vi "Disable Radio Buttons.vi"(10 "Array in":variant[](array[variant]), 11 "Controls[]":refnum<vi>[](array[refnum])) -> (3 "Array out":i32[](array[numeric]))   [LabVIEW 2020]
panel:
  out "error out":errorcluster
  in  "error in (no error)":errorcluster
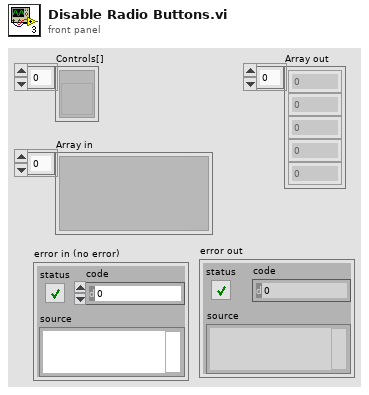
[diagram p1: front panel]
types:
  T1 = enum8{"Enabled", "Disabled", "Disabled and Grayed Out"}
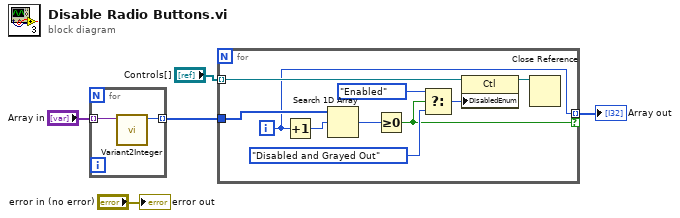
[diagram p0: block diagram]
diagram:
  n1 = for {
    tunnel: [w7] -> w3 mode=indexing
    tunnel: "Array in" -> [w6] mode=indexing
    n2 = call "Variant2Integer.vi"("Variant"=w6) -> ("data"=w7:i32)  [unwired: 9 in, 1 out]
  }
  n3 = for {
    tunnel: "Controls[]" -> [w15] mode=indexing
    tunnel: w3 -> [w17]
    tunnel: [w10] -> w5 mode=indexing if=w9
    i -> [w10]
    n4 = Increment(x=w10) -> (x+1=w8:i32)
    n5 = Search 1D Array(1D array=w17, element=w8) -> (index of element=w16:i32)  [unwired: 1 in]
    n6 = Greater Or Equal To 0?(x=w16) -> (x >= 0?=w9:bool)
    n7 = Select(t=T1."Enabled" ("Disabled"), s=w9, f=T1."Disabled and Grayed Out" ("Disabled")) -> (s? t:f=w12:T1)
    n8 = property class="Ctl"(reference=w15, "DisabledEnum"=w12) -> (reference out=w14:refnum<vi>)  [unwired: 1 in, 1 out]
    n9 = Close Reference(reference=w14) -> ()  [unwired: 1 in, 1 out]
  }
  "Array out" <- w5
  "error out" <- "error in (no error)"
